vi "Custom Freq Multiplier 3.vi"(7 "Number of pulses":u32=5, 10 "Reset":bool) -> (0 "DO State":bool, 1 "Toggle Iterations":u32, 2 "Time elapsed (ticks)":u32, 3 "FIFO Read Timed Out?":bool)   [LabVIEW 2014]
doc: "This VI is a consumer for the FIFO. The FIFO will return the dt needed for pulse high time and low time.\n\nThis VI has 2 functions.\nIf FIFO element is pos, it will generate pulse according to dt from FIFO and \"Number of pulse\" input.\nIf FIFO element is neg, it will delay according to dt from FIFO."
uses:
  Custom Pulse 2.ctl
  <vilib>/rvi/Emulation/niFpgaEmulationIsFPGAContextNoSignature.vi
  <vilib>/rvi/Emulation/niFpgaSctlEmulationGetInTimedLoop.vi
  <vilib>/rvi/errors/niFpgaSetErrorForExecOnDevCompSimple.vi
  <vilib>/rvi/eio/common/nirviEmuReportErrorAndStop.vi
  <vilib>/rvi/DataTransferAndStorage/Container/Common/niFpgaContainerGetUniqueNameForEmu.vi
  <vilib>/rvi/FIFO/Fifo_Resource/nirvififoEmulationSetSize.vi
  <vilib>/rvi/FIFO/Fifo_Resource/nirviFifoEmulationQueueMgr.vi
  <instcachedir>/0/nirviFifoEmulationQueueMgr_E5CAEC123FF24DC58D834DCA3CDAA9B5.lvgen/nirviFifoEmulationQueueMgr_E5CAEC123FF24DC58D834DCA3CDAA9B5_004.vi
  <vilib>/rvi/FIFO/Fifo_Resource/nirvififoEmulationCreateLock.vi
  <vilib>/rvi/Emulation/niFpgaProcessEmulError.vi
  <vilib>/rvi/FIFO/Fifo_Resource/nirvififoEmulationObtainLock.vi
  <vilib>/rvi/FIFO/Fifo_Resource/nirvififoEmulationReleaseLock.vi
  <vilib>/rvi/occurrence/nirviWaitOnOccurrenceBase.vi
  <vilib>/rvi/errors/nirviReportUnexpectedCaseInternalError.vi
  <vilib>/rvi/errors/nirviReportUnexpectedCaseInternalError (U32).vi
  <vilib>/rvi/DataTransferAndStorage/Container/XNode/niFpgaContainer.xnode
  <vilib>/rvi/FIFO/Fifo_Resource/nirvififoEmulationRead.vi
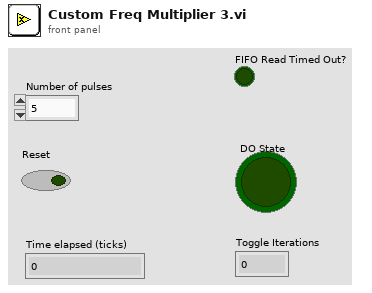
[diagram p1: front panel]
types:
  T1 = typedef "Custom Pulse 2.ctl" = enum16{"Idle", "Processing", "Delay"}
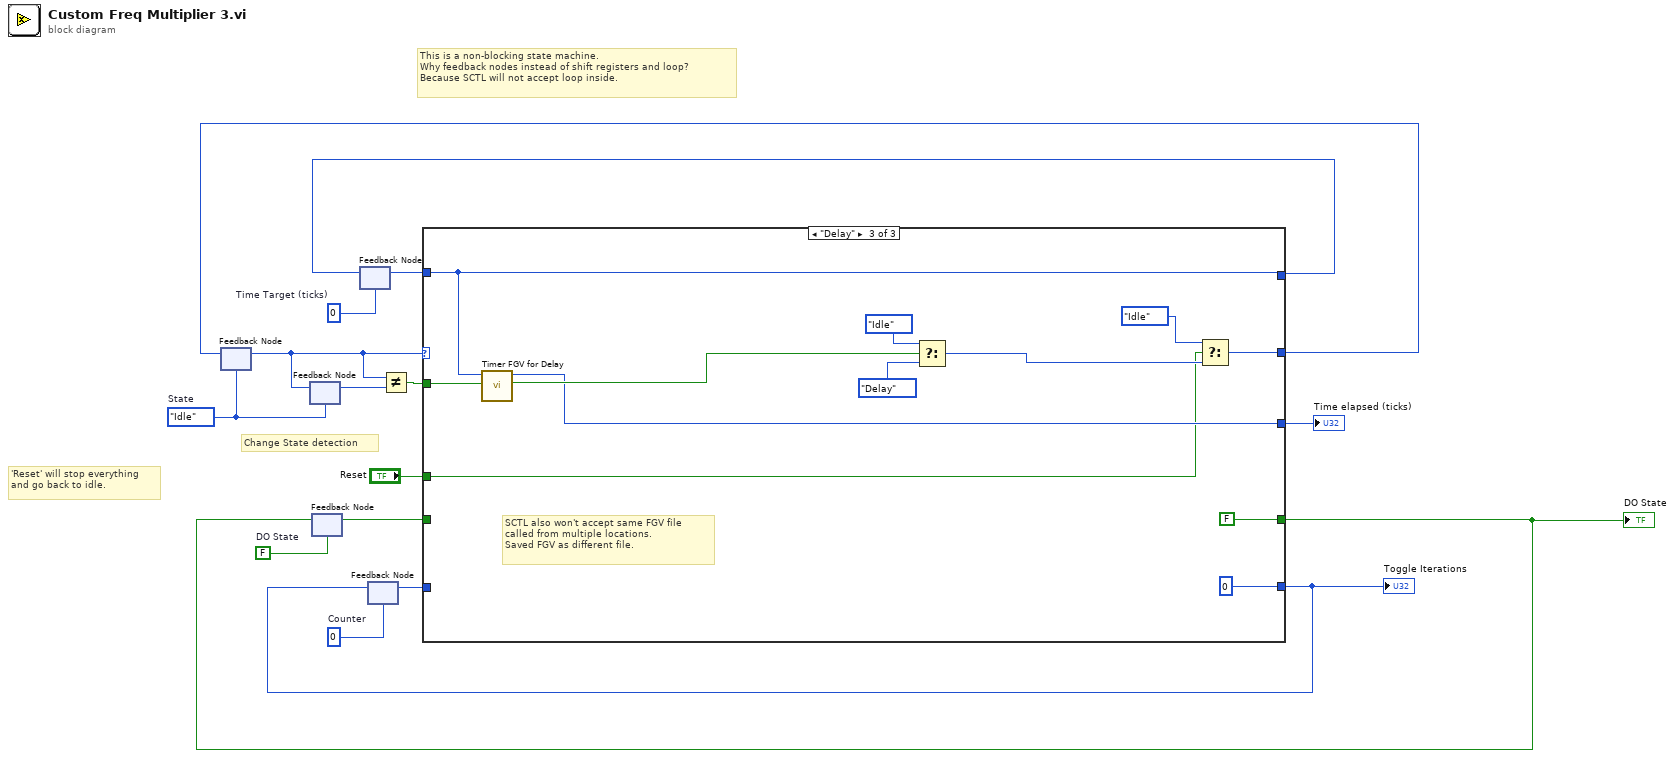
[diagram p0: block diagram]
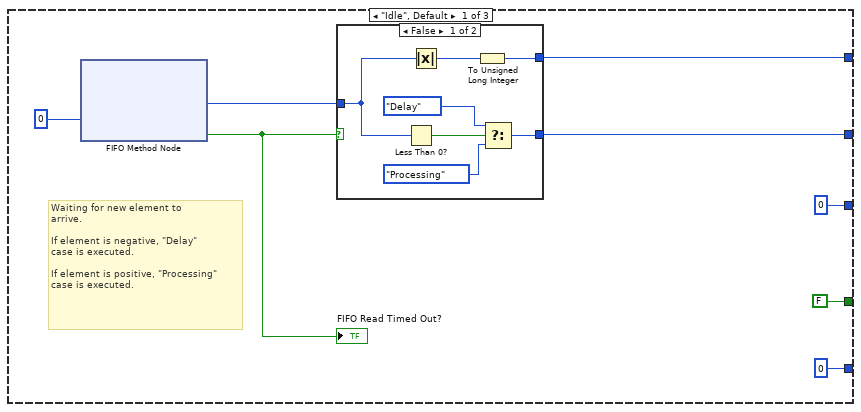
[diagram p2: hidden frame]
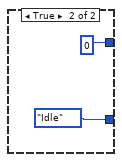
[diagram p3: hidden frame]
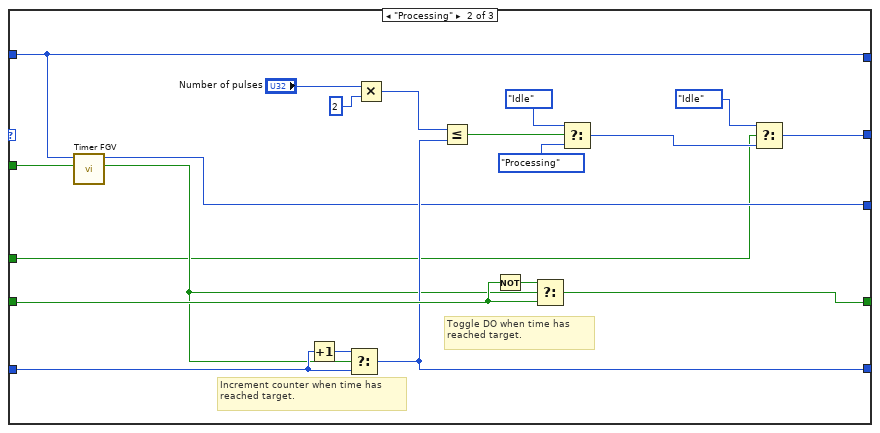
[diagram p4: hidden frame]
diagram:
  w6 = Custom_Pulse_2."Idle"  # State
  w8 = FALSE  # DO State
  w9 = u32 0  # Counter
  w10 = u32 0  # Time Target (ticks)
  # "'Reset' will stop everything\nand go back to idle."
  # "This is a non-blocking state machine.\nWhy feedback nodes instead of shift registers and loop?\nBecause SCTL will not accept loop inside."
  # "Change State detection"
  n1 = feedback #1(w6) -> (w5:T1)
  n2 = feedback #2(w6) -> (w4:T1)
  n3 = feedback-in #2(w5) -> ()
  n4 = feedback #3(w8) -> (w13:bool)
  n5 = feedback #4(w10) -> (w16:u32)
  n6 = feedback #5(w9) -> (w15:u32)
  n7 = Not Equal?(x=w5, y=w4) -> (x != y?=w3:bool)
  n8 = case shown="\"Delay\"" w5 {
    tunnel: [w17 w42 w64] -> w11
    tunnel: [w20 w35 w56] -> w7
    tunnel: w16 -> [_ w42 w64]
    tunnel: w15 -> [_ w45 _]
    tunnel: [u32 0 w43 u32 0 ("Counter")] -> w14
    tunnel: w13 -> [_ w51 _]
    tunnel: [FALSE ("DO State") w50 FALSE ("DO State")] -> w12
    tunnel: w3 -> [_ w39 w65]
    tunnel: [u32 0 ("Time elapsed (ticks)") w38 w58] -> w2
    tunnel: "Reset" -> [_ w34 w54]
    frame "Idle", Default {
      # "Waiting for new element to\narrive.\n\nIf element is negative, \"Delay\"\ncase is executed.\n\nIf element is positive, \"Processing\"\ncase is executed."
      n9 = xnode ("FIFO Method Node")("Timeout"=0) -> ("Element"=w18:i32, "Timed Out?"=w21:bool)  [unwired: 1 in, 1 out]
      "FIFO Read Timed Out?" <- w21
      n10 = case shown="False" w21 {
        tunnel: [w31 Custom_Pulse_2."Idle"] -> w20
        tunnel: w18 -> [w27 _]
        tunnel: [w25 u32 0 ("Element")] -> w17
        frame False {
          n11 = Less Than 0?(x=w27) -> (x < 0?=w28:bool)
          n12 = Absolute Value(x=w27) -> (abs(x)=w26:i32)
          n13 = To Unsigned Long Integer(number=w26) -> (unsigned 32bit integer=w25:u32)
          n14 = Select(t=Custom_Pulse_2."Delay", s=w28, f=Custom_Pulse_2."Processing") -> (s? t:f=w31:T1)
        }
        frame True {
        }
      }
    }
    frame "Processing" {
      # "Increment counter when time has\nreached target."
      # "Toggle DO when time has\nreached target."
      n15 = call "Timer FGV.vi"("Reset"=w39, "Time Target (ticks)"=w42) -> ("Time Reached?"=w41:bool, "Time elapsed (ticks)"=w38:u32)  [unwired: 8 in]
      n16 = Increment(x=w45) -> (x+1=w53:u32)
      n17 = Select(t=w53, s=w41, f=w45) -> (s? t:f=w43:u32)
      n18 = Multiply(x="Number of pulses", y=u32 2) -> (x*y=w44:u32)
      n19 = Less Or Equal?(x=w44, y=w43) -> (x <= y?=w47:bool)
      n20 = Not(x=w51) -> (.not. x?=w52:bool)
      n21 = Select(t=w52, s=w41, f=w51) -> (s? t:f=w50:bool)
      n22 = Select(t=Custom_Pulse_2."Idle", s=w47, f=Custom_Pulse_2."Processing") -> (s? t:f=w36:T1)
      n23 = Select(t=Custom_Pulse_2."Idle", s=w34, f=w36) -> (s? t:f=w35:T1)
    }
    frame "Delay" {
      # "SCTL also won't accept same FGV file\ncalled from multiple locations.\nSaved FGV as different file."
      n24 = call "Timer FGV for Delay.vi"("Reset"=w65, "Time Target (ticks)"=w64) -> ("Time Reached?"=w61:bool, "Time elapsed (ticks)"=w58:u32)  [unwired: 8 in]
      n25 = Select(t=Custom_Pulse_2."Idle", s=w61, f=Custom_Pulse_2."Delay") -> (s? t:f=w55:T1)
      n26 = Select(t=Custom_Pulse_2."Idle", s=w54, f=w55) -> (s? t:f=w56:T1)
    }
  }
  "Toggle Iterations" <- w14
  "DO State" <- w12
  "Time elapsed (ticks)" <- w2
  n27 = feedback-in #1(w7) -> ()
  n28 = feedback-in #3(w12) -> ()
  n29 = feedback-in #4(w11) -> ()
  n30 = feedback-in #5(w14) -> ()
